vi "Get FP By Name.vi"(8 "error in (no error)":errorcluster, 11 "WFP Name":string) -> (0 "error out":errorcluster, 2 "Found":bool, 3 "Web FP Out":refnum<class "Web Front Panel.lvclass">)   [LabVIEW 2016, in "Front Panel Publisher.lvlib" / "Front Panel Manager.lvclass"]
uses:
  Front Panel Manager.lvclass
  Web Front Panel_class/Web Front Panel.lvclass
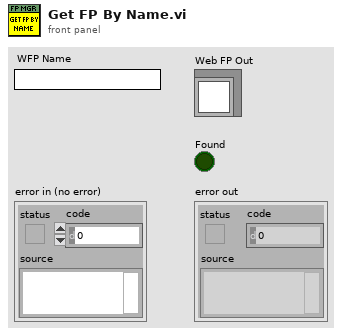
[diagram p1: front panel]
types:
  T1 = typedef "Front Panel Publisher.lvlib/Front Panel Manager.lvclass/Object Attributes.ctl" = cluster{"WebFrontPanels":refnum<class "Web Front Panel.lvclass">[], "WFP Names":string[], "Root folder":path, "Websocket Info":T2}
  T2 = typedef "Front Panel Publisher.lvlib/Front Panel Manager.lvclass/Websocket Info.ctl" = cluster{"Hostname":string, "Port":u16}
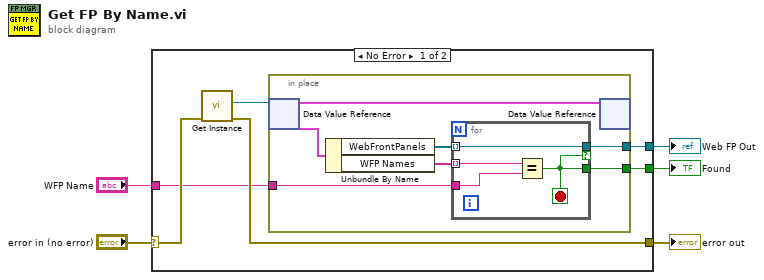
[diagram p0: block diagram]
diagram:
  n1 = case shown="No Error" "error in (no error)" {
    selector: "error in (no error)" -> [w11 w22]
    tunnel: [w10 w22] -> w4
    tunnel: "WFP Name" -> [w8 _]
    tunnel: [w7 _] -> w2
    tunnel: [w6 _] -> w1
    frame No Error {
      n2 = call "Get Instance.vi"("error in (no error)"=w11) -> ("error out"=w10:errorcluster, "DVRRefOut"=w9:refnum<data-value>)  [unwired: 6 in, 3 out]
      n3 = in-place {
        in-place-border: w8 -> [w14]
        in-place-border: [w13] -> w7
        in-place-border: [w12] -> w6
        n4 = in-place-dvr #1(w9) -> (w17:T1)  [unwired: 1 out]
        n5 = Unbundle By Name(w17) -> ("WebFrontPanels"=w16:refnum<class "Web Front Panel.lvclass">[], "WFP Names"=w15:string[])
        n6 = for {
          tunnel: w16 -> [w19] mode=indexing
          tunnel: w15 -> [w21] mode=indexing
          tunnel: w14 -> [w20]
          tunnel: [w19] -> w13 if=w18
          tunnel: [w18] -> w12
          stop <- w18 stop-if-true
          n7 = Equal?(x=w21, y=w20) -> (x = y?=w18:bool)
        }
        n8 = in-place-dvr #1(w17) -> ()  [unwired: 2 out]
      }
    }
    frame Error {
    }
  }
  "error out" <- w4
  "Web FP Out" <- w2
  "Found" <- w1
